vi "Base Serial Class Tester.vi"() -> ()   [LabVIEW 2022 SP3]
uses:
  Serial Base Class/Object Argument--cluster.ctl
  Serial Base Class/Termination Character--enum.ctl
  Serial Base Class/Serial Base.lvclass
panel:
  in  "stop":bool
  out "bytes sent":u32
  in  "Termination Char":T1=enum."\\r\\n"
  in  "pre-read delay":i16=-1
  out "bytes out count":u32
  in  "Serial Config":T2={"Com Port"="", "baud rate"=0, "data bits"=8, "parity"=enum."None", "timeout "=10000} {"data bits" min=5 max=8 step=1}
  out "Buffer Out":string
  in  "Data Command":string
  in  "Send":bool
  in  "Send Line":bool
  in  "Send and Receive":bool
  in  "Read Buffer":bool
  in  "Close":bool
  in  "Open":bool
  in  "Init":bool
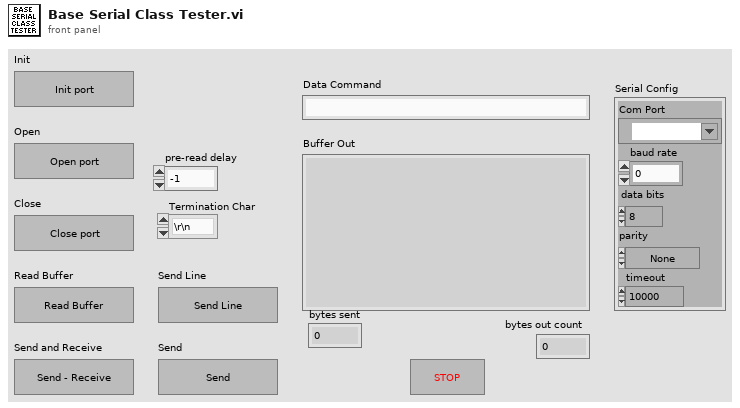
[diagram p1: front panel]
types:
  T1 = typedef "Serial Base.lvclass/Termination Character--enum.ctl" = enum16{"none", "\\r\\n", "\\r", "\\n"}
  T2 = typedef "Serial Base.lvclass/Object Argument--cluster.ctl" = cluster{"Com Port":refnum<visa-resource-name>, "baud rate":u32, "data bits":u16, "parity":enum16{"None", "Odd", "Even", "Mark", "Space"}, "timeout ":u32}
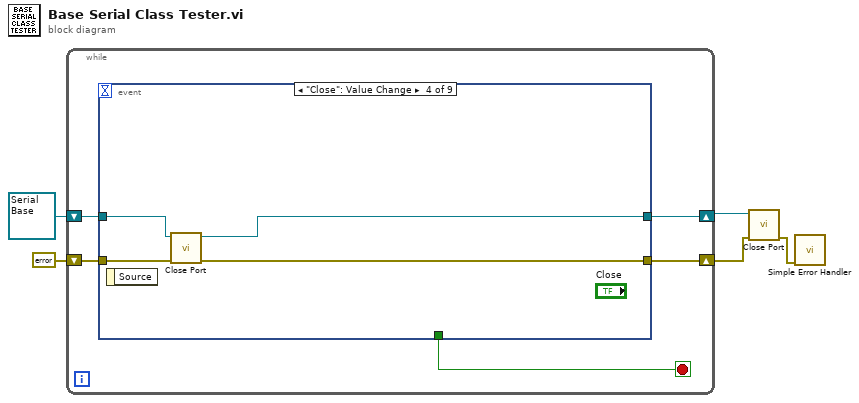
[diagram p0: block diagram]
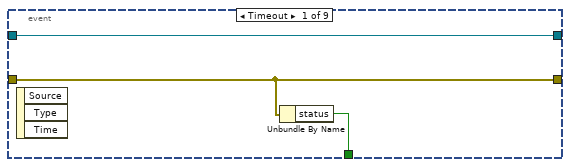
[diagram p2: hidden frame]
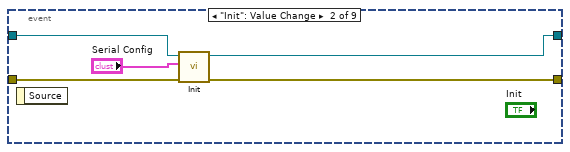
[diagram p3: hidden frame]
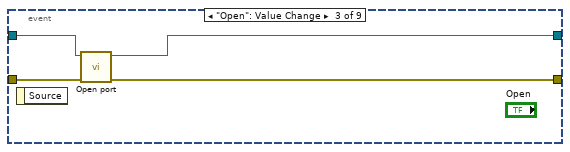
[diagram p4: hidden frame]
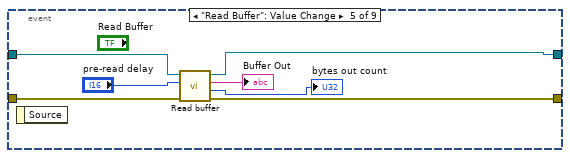
[diagram p5: hidden frame]
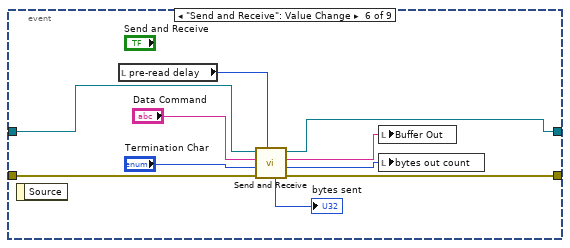
[diagram p6: hidden frame]
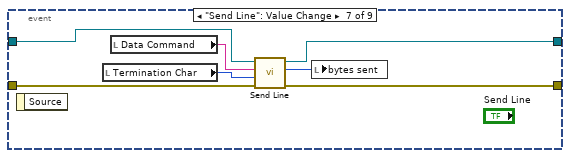
[diagram p7: hidden frame]
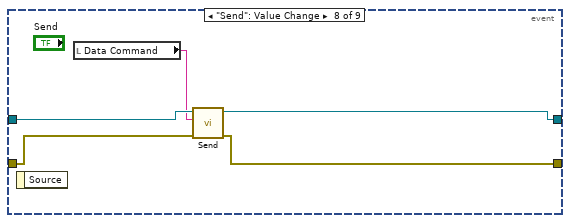
[diagram p8: hidden frame]
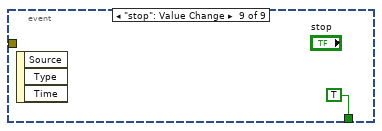
[diagram p9: hidden frame]
diagram:
  n1 = while {
    shift-right: [w8] -> w3
    shift-left: refnum<class "Serial Base.lvclass"> refnum ("Serial Base in") -> [w9]
    shift-right: [w7] -> w2
    shift-left: errorcluster {"status"=FALSE, "code"=0, "source"=""} ("error in (no error)") -> [w10]
    stop <- w6 stop-if-true
    n2 = event shown="[3] \"Close\": Value Change" {
      selector: _ -> [_ _ _ _ _ _ _ _ _]
      dyn-events: _ -> [_ _ _ _ _ _ _ _ _]
      timeout: _ -> [_ _ _ _ _ _ _ _ _]
      tunnel: w10 -> [w12 w18 w21 w25 w32 w38 w49 w54 _]
      tunnel: w9 -> [w13 w17 w22 w26 w33 w43 w50 w55 _]
      tunnel: [w13 w16 w20 w24 w30 w42 w47 w52 _] -> w8
      tunnel: [w12 w15 w19 w23 w31 w39 w48 w53 _] -> w7
      tunnel: [w11 _ _ _ _ _ _ _ TRUE] -> w6
      event Timeout {
        n3 = event-data() -> ()  [unwired: 1 in, 3 out]
        n4 = Unbundle By Name(w12) -> ("status"=w11:bool)
      }
      event "Init": Value Change {
        n5 = event-data() -> ()  [unwired: 1 in, 1 out]
        n6 = call-dynamic "Init.vi"("error in (no error)"=w18, "Serial Config"="Serial Config", "Serial Base in"=w17) -> ("error out"=w15:errorcluster, "Serial Base out"=w16:refnum<class "Serial Base.lvclass">)  [unwired: 7 in]
      }
      event "Open": Value Change {
        n7 = event-data() -> ()  [unwired: 1 in, 1 out]
        n8 = call-dynamic "Open port.vi"("error in (no error)"=w21, "Serial Base in"=w22) -> ("error out"=w19:errorcluster, "Serial Base out"=w20:refnum<class "Serial Base.lvclass">)  [unwired: 8 in]
      }
      event "Close": Value Change {
        n9 = event-data() -> ()  [unwired: 1 in, 1 out]
        n10 = call-dynamic "Close Port.vi"("error in (no error)"=w25, "Serial Base in"=w26) -> ("error out"=w23:errorcluster, "Serial Base out"=w24:refnum<class "Serial Base.lvclass">)  [unwired: 8 in]
      }
      event "Read Buffer": Value Change {
        n11 = event-data() -> ()  [unwired: 1 in, 1 out]
        n12 = call-dynamic "Read buffer.vi"("error in (no error)"=w32, "pre-read delay"="pre-read delay", "Serial Base in"=w33) -> ("error out"=w31:errorcluster, "return count"=→"bytes out count":u32, "buffer output"=→"Buffer Out":string, "Serial Base out"=w30:refnum<class "Serial Base.lvclass">)  [unwired: 5 in]
      }
      event "Send and Receive": Value Change {
        n13 = event-data() -> ()  [unwired: 1 in, 1 out]
        n14 = local read "pre-read delay"() -> (w35:i16)
        n15 = call-dynamic "Send and Receive.vi"("pre-read delay"=w35, "error in (no error)"=w38, "Termination Char"="Termination Char", "data"="Data Command", "Serial Base in"=w43) -> ("error out"=w39:errorcluster, "bytes received"=w40:u32, "buffer output"=w41:string, "Serial Base out"=w42:refnum<class "Serial Base.lvclass">, "bytes sent"=→"bytes sent":u32)  [unwired: 2 in]
        n16 = local write "Buffer Out"(w41) -> ()
        n17 = local write "bytes out count"(w40) -> ()
      }
      event "Send Line": Value Change {
        n18 = event-data() -> ()  [unwired: 1 in, 1 out]
        n19 = local read "Termination Char"() -> (w45:T1)
        n20 = local read "Data Command"() -> (w44:string)
        n21 = call-dynamic "Send Line.vi"("error in (no error)"=w49, "Termination Char"=w45, "data"=w44, "Serial Base in"=w50) -> ("error out"=w48:errorcluster, "bytes count"=w46:u32, "Serial Base out"=w47:refnum<class "Serial Base.lvclass">)  [unwired: 5 in]
        n22 = local write "bytes sent"(w46) -> ()
      }
      event "Send": Value Change {
        n23 = event-data() -> ()  [unwired: 1 in, 1 out]
        n24 = local read "Data Command"() -> (w51:string)
        n25 = call-dynamic "Send.vi"("error in (no error)"=w54, "data"=w51, "Serial Base in"=w55) -> ("error out"=w53:errorcluster, "Serial Base out"=w52:refnum<class "Serial Base.lvclass">)  [unwired: 6 in, 1 out]
      }
      event "stop": Value Change {
        n26 = event-data() -> ()  [unwired: 1 in, 3 out]
      }
    }
  }
  n27 = call-dynamic "Close Port.vi"("error in (no error)"=w2, "Serial Base in"=w3) -> ("error out"=w1:errorcluster)  [unwired: 8 in, 1 out]
  n28 = call <vilib>:"Simple Error Handler.vi"("error in (no error)"=w1) -> ()  [unwired: 4 in, 5 out]
